vi "distance_to_voltage(SubVI).vi"(11 "distance(cm)":dbl) -> (3 "Voltage(V)":dbl)   [LabVIEW 2019]
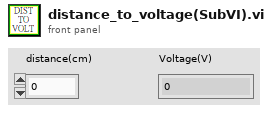
[diagram p1: front panel]
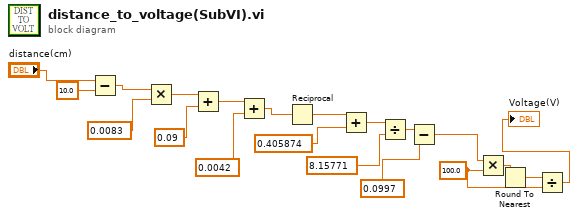
[diagram p0: block diagram]
diagram:
  w3 = 100.0 ("y")
  n1 = Subtract(x="distance(cm)", y=10.0) -> (x-y=w8:dbl)
  n2 = Multiply(x=w8, y=0.0083) -> (x*y=w10:dbl)
  n3 = Add(x=w10, y=0.09) -> (x+y=w12:dbl)
  n4 = Add(x=w12, y=0.0042) -> (x+y=w14:dbl)
  n5 = Reciprocal(x=w14) -> (1/x=w15:dbl)
  n6 = Add(x=w15, y=0.405874) -> (x+y=w17:dbl)
  n7 = Divide(x=w17, y=8.15771 ("m")) -> (x/y=w19:dbl)
  n8 = Subtract(x=w19, y=0.0997) -> (x-y=w5:dbl)
  n9 = Multiply(x=w5, y=w3) -> (x*y=w4:dbl)
  n10 = Round To Nearest(number=w4) -> (nearest integer value=w1:dbl)
  n11 = Divide(x=w1, y=w3) -> (x/y=→"Voltage(V)":dbl)
